vi "FinalSansReference.vi"() -> ()   [LabVIEW 2013]
uses:
  <vilib>/DAQmx/read.llb/DAQmx Read (Analog Wfm 1Chan NSamp).vi
  <vilib>/DAQmx/miscellaneous.llb/DAQmx Fill In Error Info.vi
  <vilib>/express/express analysis/Spectral/Block/exnSpectralBlock spectral measurements PSD poly.vi
  <vilib>/express/express analysis/Spectral/Block/exnSpectralBlock spectral measurements PSD WFM.vi
  <vilib>/express/express analysis/Spectral/XNode/ExpressSpectralMeasurementsBlockNode.xnode
panel:
  in  "Voie physique DAQmx":tag="sHIT/ai0"
  in  "Statistiques":bool
  out "Moyenne":dbl
  out "Valeur eff":dbl
  out "Frequence":dbl
  in  "FFT":bool
  in  "Fenetre d'affichage (s)":dbl step=0.001
  out "Signal":waveform(dbl)(graph)
  out "FFT":cluster{"f0":dbl, "df":dbl, "magnitude":dbl[]}(graph)
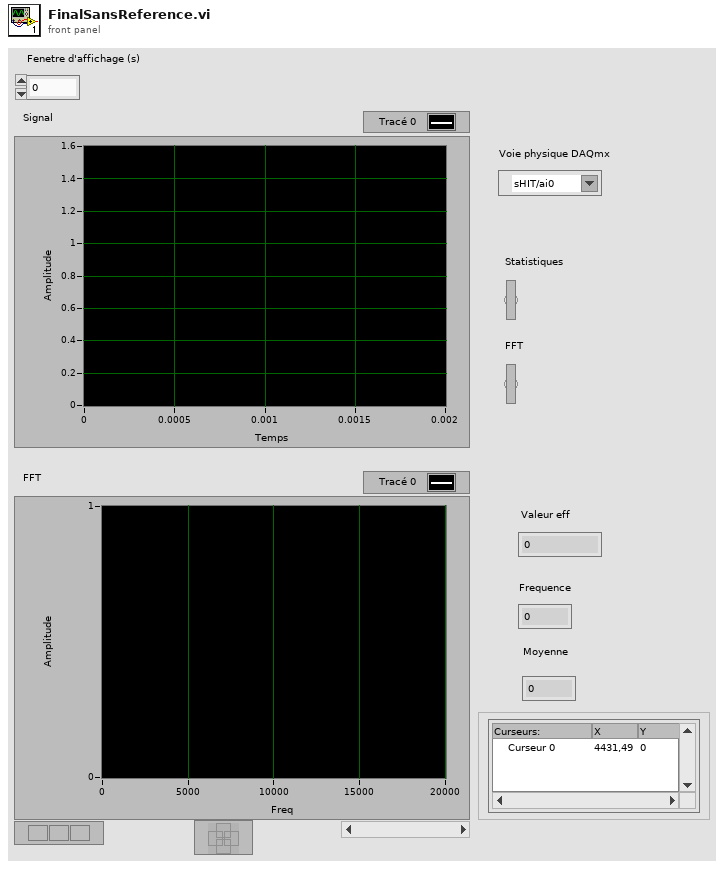
[diagram p1: front panel]
types:
  T1 = cluster{"averaging mode":u16, "weighting mode":u16, "number of averages":u32}
  T2 = cluster{"dB On (F)":bool, "unwrap phase (F)":bool, "convert to degree (F)":bool}
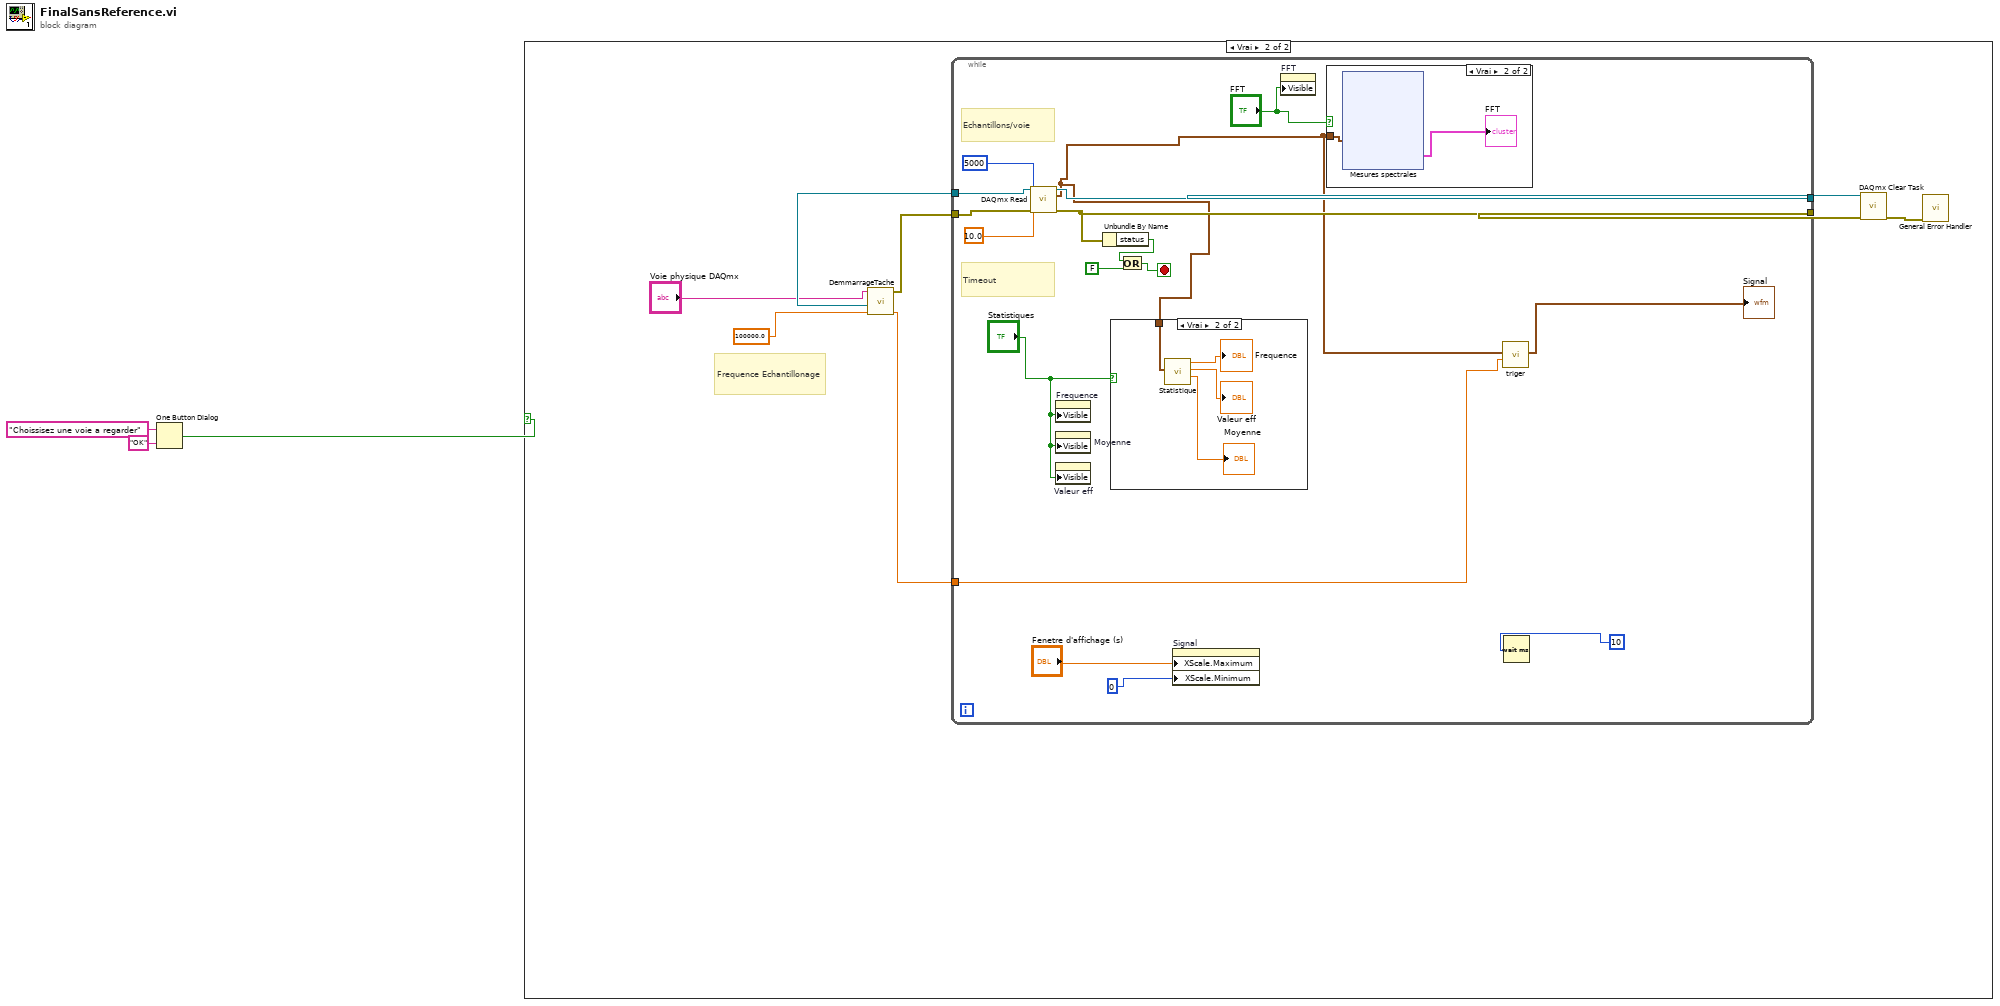
[diagram p0: block diagram]
diagram:
  n1 = One Button Dialog(message="Choissisez une voie a regarder", button name ("OK")="OK" ("nom du bouton (\"OK\")")) -> (true=w1:bool)
  n2 = case shown="Vrai" w1 {
    frame False {
    }
    frame True {
      # "Frequence Echantillonage"
      n3 = call "DemmarrageTache.vi"("frequence echantillonage"=100000.0, "Voie physique DAQmx"="Voie physique DAQmx") -> ("frequence echantillonage 2"=w5:dbl, "task out"=w6:refnum<k21>, "error out"=w7:errorcluster)  [unwired: 6 in]
      n4 = while {
        tunnel: w6 -> [w28]
        tunnel: w7 -> [w27]
        tunnel: [w25] -> w11
        tunnel: [w21] -> w10
        tunnel: w5 -> [w13]
        stop <- w24 stop-if-true
        # "Echantillons/voie"
        # "Timeout"
        n5 = call-poly <vilib>:"DAQmx Read.vi"("task/channels in"=w28, "number of samples per channel"=5000, "timeout"=10.0, "error in"=w27) -> ("task out"=w25:refnum<k21>, "data"=w14:waveform(dbl), "error out"=w21:errorcluster)  [unwired: 9 in]
        n6 = property on="Frequence" class="NumNb (strict)"("Visible"="Statistiques") -> ()  [unwired: 2 in, 2 out]
        n7 = property on="Moyenne" class="NumNb (strict)"("Visible"="Statistiques") -> ()  [unwired: 2 in, 2 out]
        n8 = property on="Valeur eff" class="NumNb (strict)"("Visible"="Statistiques") -> ()  [unwired: 2 in, 2 out]
        n9 = Unbundle By Name(w21) -> ("status"=w22:bool)
        n10 = case shown="Vrai" "Statistiques" {
          tunnel: w14 -> [_ w32]
          frame False {
          }
          frame True {
            n11 = call "Statistique.vi"("Waveform"=w32) -> ("mean"=→"Moyenne":dbl, "Valeur efficace"=→"Valeur eff":dbl, "Fréquence"=→"Frequence":dbl)  [unwired: 8 in]
          }
        }
        n12 = Or(x=w22, y=FALSE) -> (x .or. y?=w24:bool)
        n13 = property on="Signal" class="GraphWF (strict)"("XScale.Maximum"="Fenetre d'affichage (s)", "XScale.Minimum"=0) -> ()  [unwired: 2 in, 2 out]
        n14 = property on="FFT" class="GraphWF (strict)"("Visible"="FFT") -> ()  [unwired: 2 in, 2 out]
        n15 = case shown="Vrai" "FFT" {
          tunnel: w14 -> [_ w33]
          frame False {
          }
          frame True {
            n16 = xnode "Mesures spectrales"("Signaux"=w33) -> ("DSP"=→"FFT":cluster{"f0":dbl, "df":dbl, "magnitude":dbl[]})  [unwired: 1 in, 1 out]
          }
        }
        n17 = call "triger.vi"("frequene echantillonage"=w13, "Signal"=w14) -> ("waveform en sortie"=→"Signal":waveform(dbl))  [unwired: 9 in]
        n18 = Wait (ms)(milliseconds to wait=10) -> ()  [unwired: 1 out]
      }
      n19 = call <vilib>:"DAQmx Clear Task.vi"("task in"=w11, "error in"=w10) -> ("error out"=w9:errorcluster)  [unwired: 13 in]
      n20 = call <vilib>:"General Error Handler.vi"("error in (no error)"=w9) -> ()  [unwired: 10 in, 5 out]
    }
  }
